vi "LED_Brightnes.vi"(8 "error in (no error)":errorcluster, 10 "LEDParam":T1={"Period"=1000, "DutyCycle"=0, "LED#"="/led1"}, 11 "FPGA VI":refnum<k20>) -> (0 "error out":errorcluster, 3 "FPGA VI Reference Out":refnum<k20>)   [LabVIEW 2015]
uses:
  <vilib>/Utility/error.llb/Error Cluster From Error Code.vi
  <vilib>/rvi/errors/niLvFpgaAdjustHostInterfaceError.vi
  <vilib>/rvi/interface/nirviReadWriteControl/nirviReadWriteControl.xnode
  NiFpgaLv.dll
  <vilib>/rvi/interface/Simulation/niFpgaSimulationCallBeginRW.vi
panel:
  in  "LEDParam":T2
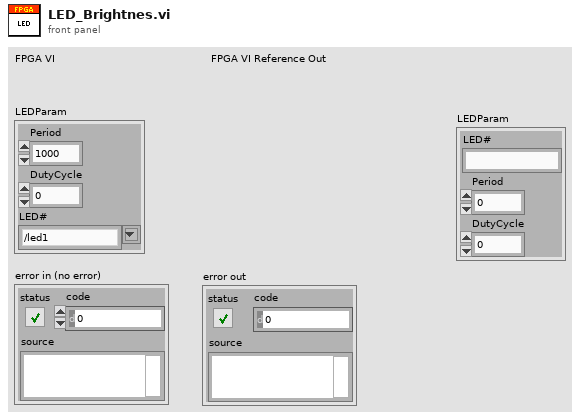
[diagram p1: front panel]
types:
  T1 = cluster{"Period":u32, "DutyCycle":u32, "LED#":string}
  T2 = cluster{"LED#":string, "Period":u32, "DutyCycle":u32}
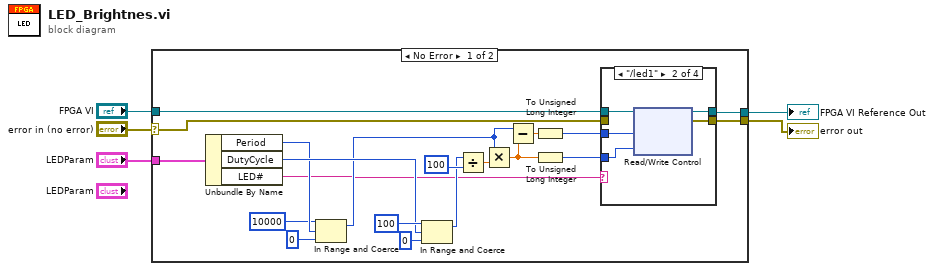
[diagram p0: block diagram]
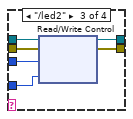
[diagram p3: hidden frame]
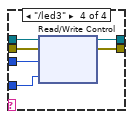
[diagram p4: hidden frame]
diagram:
  n1 = case shown="No Error" "error in (no error)" {
    selector: "error in (no error)" -> [w6 w45]
    tunnel: [w21 w46] -> w5
    tunnel: "FPGA VI" -> [w20 w46]
    tunnel: [w19 w45] -> w3
    tunnel: "LEDParam" -> [w7 _]
    frame No Error {
      n2 = Unbundle By Name(w7) -> ("Period"=w12:u32, "DutyCycle"=w14:u32, "LED#"=w8:string)
      n3 = In Range and Coerce(upper limit=u32 10000, x=w12, lower limit=u32 0) -> (coerced(x)=w11:u32)  [unwired: 1 out]
      n4 = In Range and Coerce(upper limit=100, x=w14, lower limit=0) -> (coerced(x)=w13:u32)  [unwired: 1 out]
      n5 = Divide(x=w13, y=100) -> (x/y=w23:dbl)
      n6 = Multiply(x=w11, y=w23) -> (x*y=w25:dbl)
      n7 = Subtract(x=w11, y=w25) -> (x-y=w24:dbl)
      n8 = To Unsigned Long Integer(number=w24) -> (unsigned 32bit integer=w18:u32)
      n9 = To Unsigned Long Integer(number=w25) -> (unsigned 32bit integer=w17:u32)
      n10 = case shown="\"/led1\"" w8 {
        tunnel: [w27 w29 w35 w41] -> w21
        tunnel: w20 -> [w27 w32 w38 w44]
        tunnel: [w26 w28 w36 w42] -> w19
        tunnel: w6 -> [w26 _ w37 w43]
        tunnel: w18 -> [_ w31 w34 w40]
        tunnel: w17 -> [_ w30 w33 w39]
        frame "Default", Default {
        }
        frame "/led1" {
          n11 = xnode "Read/Write Control"("FPGA VI Reference In"=w32, "LED1_H"=w31, "LED1_L"=w30) -> ("FPGA VI Reference Out"=w29:refnum<k20>, "error out"=w28:errorcluster)  [unwired: 1 in]
        }
        frame "/led2" {
          n12 = xnode "Read/Write Control"("FPGA VI Reference In"=w38, "error in"=w37, "LED2_H"=w34, "LED2_L"=w33) -> ("FPGA VI Reference Out"=w35:refnum<k20>, "error out"=w36:errorcluster)
        }
        frame "/led3" {
          n13 = xnode "Read/Write Control"("FPGA VI Reference In"=w44, "error in"=w43, "LED3_H"=w40, "LED3_L"=w39) -> ("FPGA VI Reference Out"=w41:refnum<k20>, "error out"=w42:errorcluster)
        }
      }
    }
    frame Error {
    }
  }
  "error out" <- w3
  "FPGA VI Reference Out" <- w5
